vi "扫描参数.vi"(7 "refnum":T1 caption="引用句柄", 10 "测试人员":string, 11 "错误输入（无错误）":errorcluster) -> (2 "扫描":T2={"测试参数"={"正向电压(V)"=0.0, "正向极限电流(mA)"=0.0, "反向电压(V)"=0.0, "反向极限电流(mA)"=0.0, "电压改变量(V)"=0.0}, "时序参数"={"维持时间(ms)"=0.0, "nplc"=0.001, "时序优先"=FALSE}} {"测试参数"."反向极限电流(mA)" min=0.0 max=3000.0; "测试参数"."反向电压(V)" min=0.0 max=40.0; "测试参数"."电压改变量(V)" min=0.0 max=40.0 step=5e-06; "测试参数"."正向极限电流(mA)" min=0.0 max=3000.0; "测试参数"."正向电压(V)" min=0.0 max=40.0; "时序参数"."nplc" min=0.001}, 3 "错误输出":errorcluster, 5 "refnum out":T1 caption="引用句柄输出")   [LabVIEW 2021]
uses:
  <vilib>/Utility/config.llb/Config Data RefNum.ctl
  <vilib>/Utility/config.llb/Read Key (String).vi
  <vilib>/Utility/config.llb/NI_LVConfig.lvlib
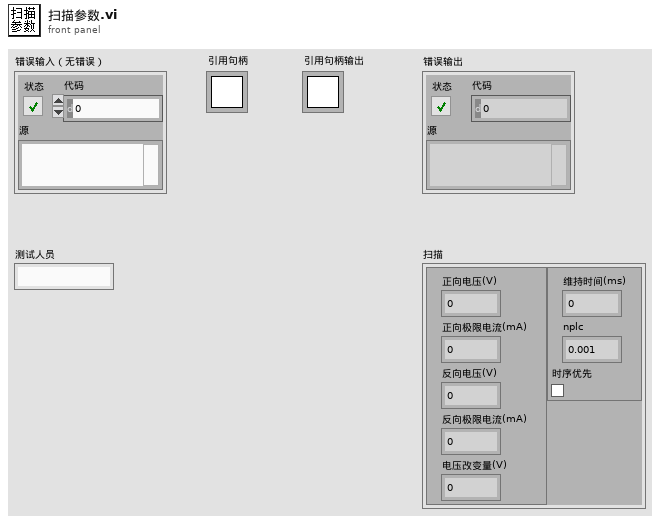
[diagram p1: front panel]
types:
  T1 = typedef "NI_LVConfig.lvlib/Config Data RefNum.ctl" = refnum<k1>
  T2 = typedef "扫描参数.ctl" = cluster{"测试参数":cluster{"正向电压(V)":dbl, "正向极限电流(mA)":dbl, "反向电压(V)":dbl, "反向极限电流(mA)":dbl, "电压改变量(V)":dbl}, "时序参数":cluster{"维持时间(ms)":dbl, "nplc":dbl, "时序优先":bool}}
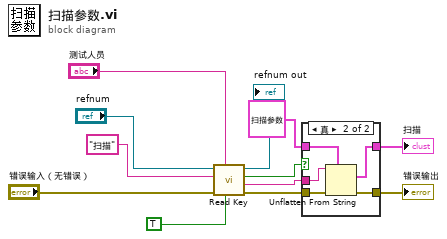
[diagram p0: block diagram]
diagram:
  n1 = call-poly <vilib>:"Read Key.vi"("read raw string? (F)"=TRUE, "section"="测试人员", "error in (no error)"="错误输入（无错误）", "key"="扫描", "refnum"="refnum") -> ("error out"=w3:errorcluster, "value"=w7:string, "found?"=w8:bool, "refnum out"=→"refnum out":T1)  [unwired: 3 in]
  n2 = case shown="真" w8 {
    tunnel: w7 -> [_ w19]
    tunnel: T2 {"测试参数"={"正向电压(V)"=1.0, "正向极限电流(mA)"=1.0, "反向电压(V)"=1.0, "反向极限电流(mA)"=1.0, "电压改变量(V)"=0.1}, "时序参数"={"维持时间(ms)"=25.0, "nplc"=0.1, "时序优先"=FALSE}} ("扫描") -> [w14 w18]
    tunnel: [w14 w17] -> w5
    tunnel: [w13 w16] -> w2
    tunnel: w3 -> [w13 w15]
    frame False {
    }
    frame True {
      n3 = Unflatten From String(type=w18, binary string=w19, error in (no error)=w15) -> (value=w17:T2, error out=w16:errorcluster)  [unwired: 2 in, 1 out]
    }
  }
  "扫描" <- w5
  "错误输出" <- w2
